vi "c_ctre_phoenix6_platform_sim_get_last_error.vi"(0 "Numeric 2":i32, 1 "Numeric 3":i32) -> (20 "Numeric":i32)   [LabVIEW 2023]
uses:
  <vilib>/Rock Robotics/WPI/ThirdParty/Phoenix-LabVIEW/Controls/DriverLib.ctl
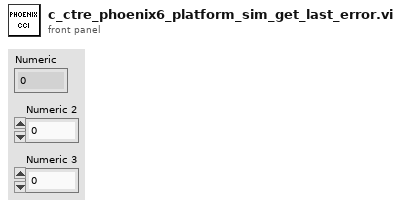
[diagram p1: front panel]
types:
  T1 = typedef "DriverLib.ctl" = path
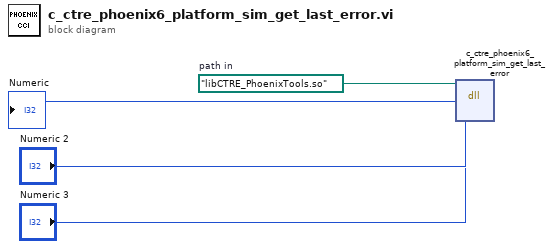
[diagram p0: block diagram]
diagram:
  w4 = T1 path "libCTRE_PhoenixTools.so"  # path in
  n1 = dll-call lib="?" fn="c_ctre_phoenix6_platform_sim_get_last_error"(path in=w4, "Numeric 2", "Numeric 3") -> (→"Numeric":i32)  [unwired: 4 in, 2 out]
